vi "act-0009-cor.vi"() -> ()   [LabVIEW 2010]
uses:
  lv_01/lv_01.lvlib
panel:
  out "valeur \nsélectionnée":dbl
  in  "sélecteur":bool
  out "Deg F":dbl format="%.2f"
  out "Deg C":dbl format="%.2f"
  # "Le sélecteur dont on change l'état affiche les degrés Celsius ou fahrenheit.\nExécutez le code chaque fosi que ous changez la valeur du sélecteur"
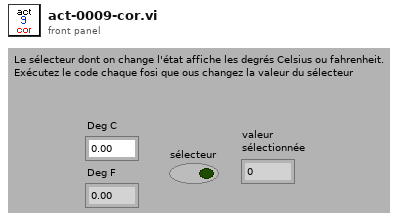
[diagram p1: front panel]
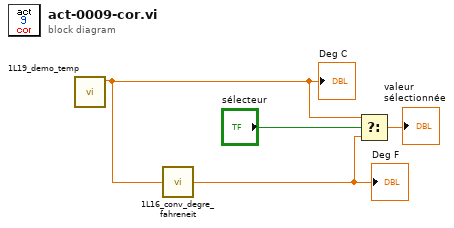
[diagram p0: block diagram]
diagram:
  n1 = call "1L19_demo_temp.vi"() -> ("temp"=w1:dbl)  [unwired: 6 in, 1 out]
  "Deg C" <- w1
  n2 = call "1L16_conv_degre_fahreneit.vi"("Deg C"=w1) -> ("Deg F"=w4:dbl)
  "Deg F" <- w4
  n3 = Select(t=w1, s="sélecteur", f=w4) -> (s? t:f=→"valeur \nsélectionnée":dbl)
